vi "Calculator.vi"() -> ()   [LabVIEW 2020]
panel:
  in  "stop":bool
  out "Answer":dbl
  in  "Y":dbl
  in  "X":dbl
  in  "Enum":T1(ring)
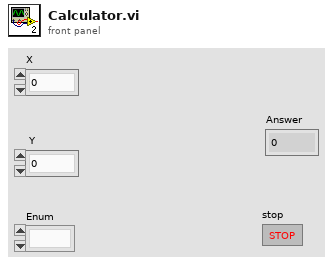
[diagram p1: front panel]
types:
  T1 = enum16{"", "Add", "Subtract", "Multiply", "Divide"}
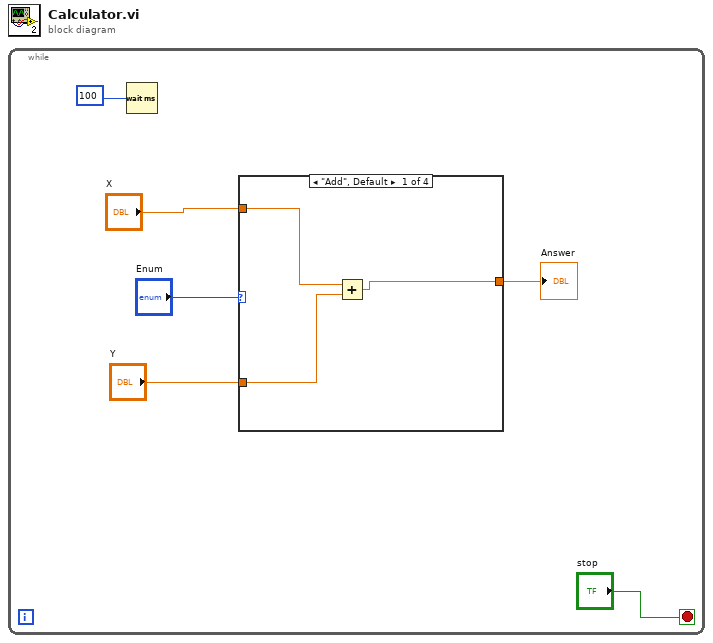
[diagram p0: block diagram]
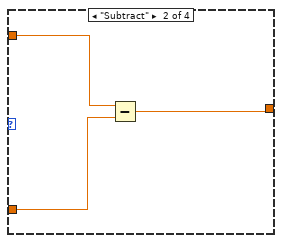
[diagram p2: hidden frame]
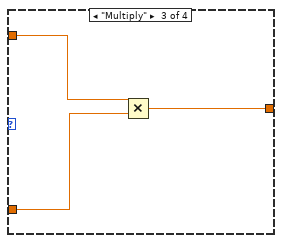
[diagram p3: hidden frame]
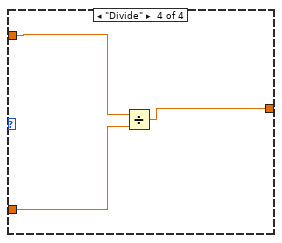
[diagram p4: hidden frame]
diagram:
  n1 = while {
    stop <- "stop" stop-if-true
    n2 = Wait (ms)(milliseconds to wait=u32 100) -> ()  [unwired: 1 out]
    n3 = case shown="\"Add\", Default" "Enum" {
      tunnel: "X" -> [w9 w12 w15 w17]
      tunnel: "Y" -> [w8 w11 w14 w18]
      tunnel: [w7 w10 w13 w16] -> w3
      frame "Add", Default {
        n4 = Add(x=w9, y=w8) -> (x+y=w7:dbl)
      }
      frame "Subtract" {
        n5 = Subtract(x=w12, y=w11) -> (x-y=w10:dbl)
      }
      frame "Multiply" {
        n6 = Multiply(x=w15, y=w14) -> (x*y=w13:dbl)
      }
      frame "Divide" {
        n7 = Divide(x=w17, y=w18) -> (x/y=w16:dbl)
      }
    }
    "Answer" <- w3
  }
